vi "BucketNearMatchingPngFiles.vi"(10 "All PNG Files":path[](array[path])) -> (3 "All PNG Files (Bucketed by Near-Matches)":cluster{"Similar PNG Files":path[]}[](array[cluster]))   [LabVIEW 2020]
panel:
  out "Image buckets":i32[](array[numeric])
  out "Report":string
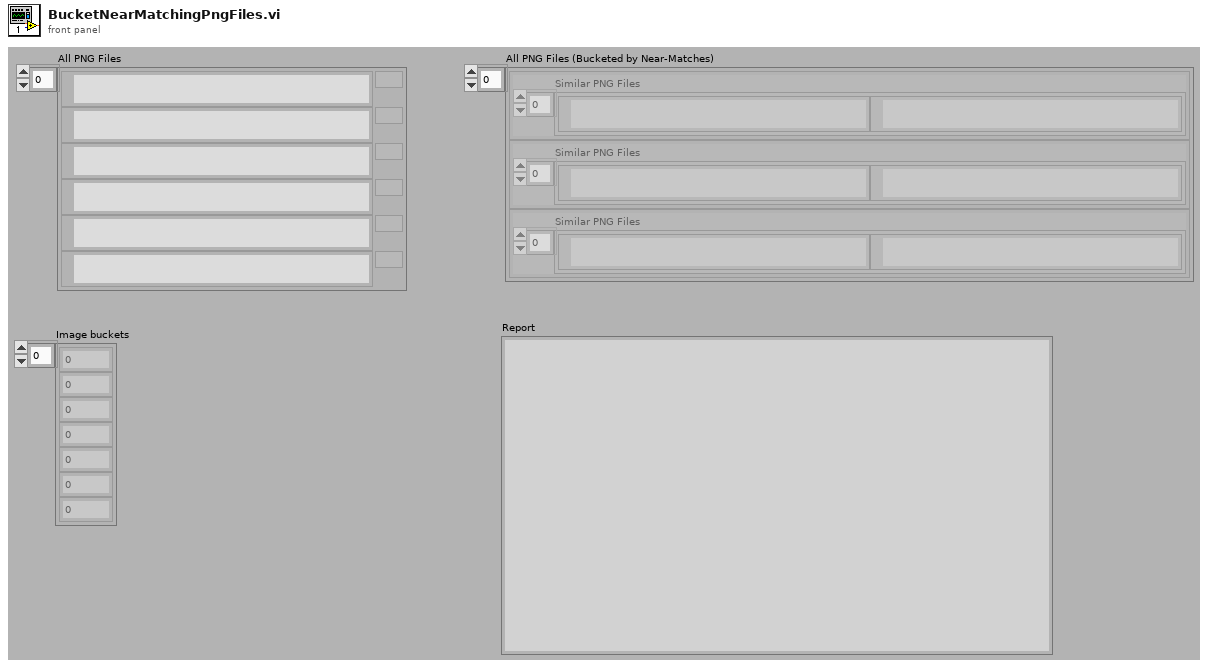
[diagram p1: front panel]
types:
  T1 = typedef "imagedata.ctl" = cluster{"image type":i32, "image depth":i32, "image":u8[], "mask":u8[], "colors":u32[], "Rectangle":cluster{"left":i16, "top":i16, "right":i16, "bottom":i16}}
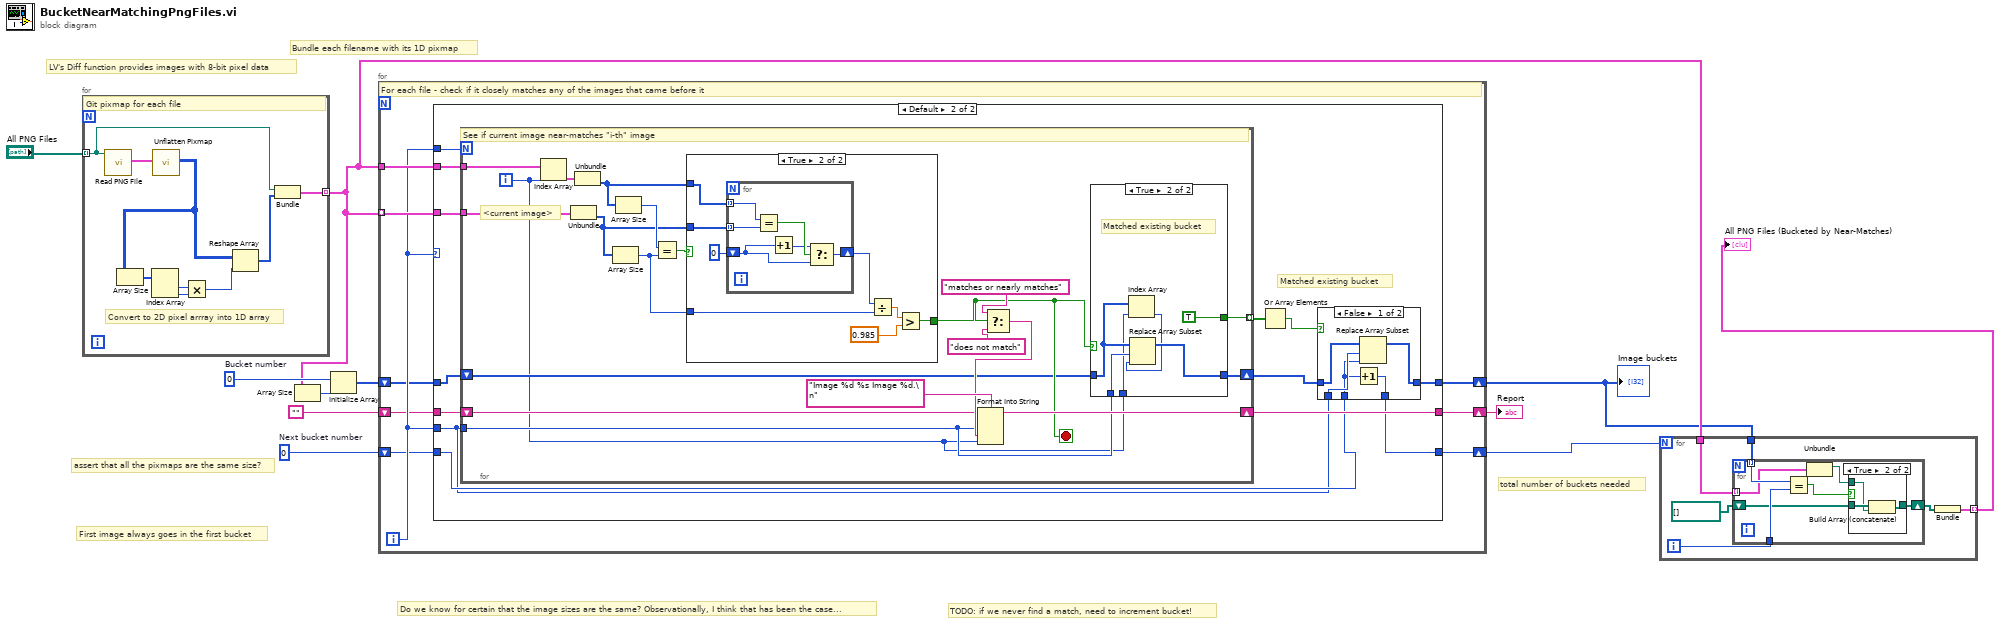
[diagram p0: block diagram]
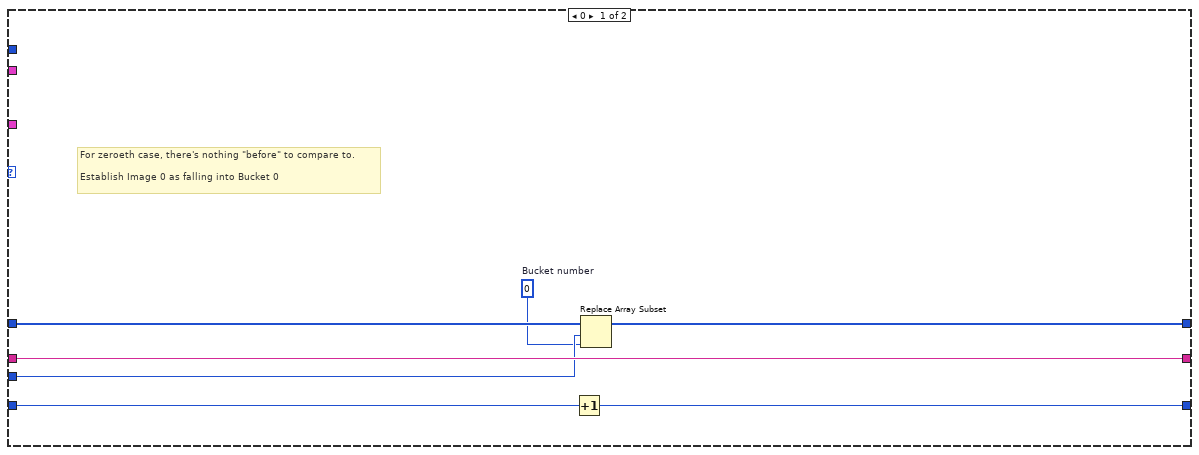
[diagram p3: hidden frame]
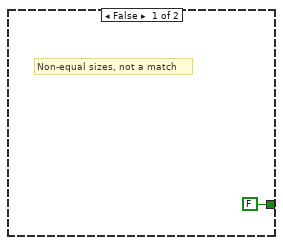
[diagram p6: hidden frame]
diagram:
  w5 = 0  # Next bucket number
  w8 = 0  # Bucket number
  # "total number of buckets needed"
  # "TODO: if we never find a match, need to increment bucket!"
  # "Do we know for certain that the image sizes are the same? Observationally, I think that has been the case..."
  # "Bundle each filename with its 1D pixmap"
  # "First image always goes in the first bucket"
  # "LV's Diff function provides images with 8-bit pixel data"
  # "assert that all the pixmaps are the same size?"
  n1 = for {
    tunnel: "All PNG Files" -> [w14] mode=indexing
    tunnel: [w12] -> w3 mode=indexing
    # "Convert to 2D pixel arrray into 1D array"
    # "Git pixmap for each file"
    n2 = call <vilib>:"Read PNG File.vi"("path to PNG file"=w14) -> ("image data"=w20:T1)  [unwired: 8 in, 2 out]
    n3 = call <vilib>:"Unflatten Pixmap.vi"("image data"=w20) -> ("8-bit pixmap"=w15:u8[][])  [unwired: 4 in, 6 out]
    n4 = Array Size(array=w15) -> (size(s)=w19:i32[])
    n5 = Index Array(array=w19) -> (element #1=w17:i32, element #2=w18:i32)  [unwired: 2 in]
    n6 = Multiply(x=w17, y=w18) -> (x*y=w16:i32)
    n7 = Reshape Array(w15, w16) -> (w13:u8[])
    n8 = Bundle("Path"=w14, "8-bit pixmap"=w13) -> (w12:cluster{"Path":path, "8-bit pixmap":u8[]})  [unwired: 1 in]
  }
  n9 = Array Size(array=w3) -> (size(s)=w7:i32)
  n10 = Initialize Array(w8, w7) -> (w6:i32[])
  n11 = for {
    tunnel: w3 -> [w29] mode=indexing
    tunnel: w3 -> [w28]
    shift-right: [w25] -> w9
    shift-left: "" -> [w26]
    shift-right: [w23] -> w2
    shift-left: w6 -> [w24]
    shift-right: [w21] -> w4
    shift-left: w5 -> [w22]
    i -> [w27]
    # "For each file - check if it closely matches any of the images that came before it"
    n12 = case shown="Default" w27 {
      tunnel: w27 -> [_ w49]
      tunnel: w29 -> [_ w48]
      tunnel: w28 -> [_ w47]
      tunnel: w27 -> [w33 w37]
      tunnel: w26 -> [w36 w46]
      tunnel: [w36 w45] -> w25
      tunnel: w24 -> [w35 w44]
      tunnel: [w34 w41] -> w23
      tunnel: w22 -> [w31 w39]
      tunnel: [w30 w38] -> w21
      frame 0 {
        w32 = 0  # Bucket number
        # "For zeroeth case, there's nothing \"before\" to compare to.\n\nEstablish Image 0 as falling into Bucket 0"
        n13 = Increment(x=w31) -> (x+1=w30:i32)
        n14 = Replace Array Subset(array=w35, new element=w32, index=w33) -> (w34:i32[])
      }
      frame Default {
        # "Matched existing bucket"
        n15 = for {
          N: w49 -> [_]
          tunnel: w48 -> [w74]
          tunnel: w47 -> [w76]
          tunnel: w37 -> [w59]
          shift-right: [w63] -> w45
          shift-left: w46 -> [w64]
          shift-right: [w60] -> w40
          shift-left: w44 -> [w61]
          tunnel: [w57] -> w43 mode=indexing
          i -> [w58]
          stop <- w62 stop-if-true
          # "<current image>"
          # "See if current image near-matches \"i-th\" image"
          n16 = Index Array(array=w76, index=w58) -> (element=w75:cluster{"Path":path, "8-bit pixmap":u8[]})
          n17 = Unbundle(w74) -> ("8-bit pixmap"=w70:u8[])  [unwired: 1 out]
          n18 = Unbundle(w75) -> ("8-bit pixmap"=w71:u8[])  [unwired: 1 out]
          n19 = Array Size(array=w70) -> (size(s)=w69:i32)
          n20 = Array Size(array=w71) -> (size(s)=w73:i32)
          n21 = Equal?(x=w73, y=w69) -> (x = y?=w72:bool)
          n22 = case shown="True" w72 {
            tunnel: w71 -> [_ w92]
            tunnel: w70 -> [_ w91]
            tunnel: w69 -> [_ w89]
            tunnel: [FALSE w85] -> w62
            frame False {
              # "Non-equal sizes, not a match"
            }
            frame True {
              n23 = for {
                tunnel: w92 -> [w97] mode=indexing
                tunnel: w91 -> [w98] mode=indexing
                shift-right: [w96] -> w88
                shift-left: 0 -> [w93]
                n24 = Equal?(x=w97, y=w98) -> (x = y?=w95:bool)
                n25 = Increment(x=w93) -> (x+1=w94:i32)
                n26 = Select(t=w94, s=w95, f=w93) -> (s? t:f=w96:i32)
              }
              n27 = Divide(x=w88, y=w89) -> (x/y=w87:dbl)
              n28 = Greater?(x=w87, y=0.985) -> (0:w85:bool)
            }
          }
          n29 = Select(t="matches or nearly matches", s=w62, f="does not match") -> (s? t:f=w65:string)
          n30 = Format Into String(format string="Image %d %s Image %d.\n", initial string=w64, w59, w65, w58) -> (resulting string=w63:string)  [unwired: 1 in, 1 out]
          n31 = case shown="True" w62 {
            tunnel: w61 -> [w77 w81]
            tunnel: [w77 w83] -> w60
            tunnel: w59 -> [_ w82]
            tunnel: w58 -> [_ w80]
            tunnel: [_ TRUE] -> w57
            frame False {
            }
            frame True {
              # "Matched existing bucket"
              n32 = Index Array(array=w81, index=w80) -> (element=w79:i32)
              n33 = Replace Array Subset(array=w81, new element=w79, index=w82) -> (w83:i32[])
            }
          }
        }
        n34 = Or Array Elements(Boolean array=w43) -> (logical OR=w42:bool)
        n35 = case shown="False" w42 {
          tunnel: [w53 w56] -> w41
          tunnel: w40 -> [w54 w56]
          tunnel: w39 -> [w51 w55]
          tunnel: [w50 w55] -> w38
          tunnel: w37 -> [w52 _]
          frame False {
            n36 = Increment(x=w51) -> (x+1=w50:i32)
            n37 = Replace Array Subset(array=w54, new element=w51, index=w52) -> (w53:i32[])
          }
          frame True {
          }
        }
      }
    }
  }
  "Report" <- w9
  "Image buckets" <- w2
  n38 = for {
    N: w4 -> [_]
    tunnel: w3 -> [w104]
    tunnel: w2 -> [w103]
    tunnel: [w99] -> w1 mode=indexing
    i -> [w102]
    n39 = for {
      tunnel: w104 -> [w109] mode=indexing
      tunnel: w103 -> [w110] mode=indexing
      tunnel: w102 -> [w111]
      shift-right: [w106] -> w100
      shift-left: path[] [] ("Similar PNG Files") -> [w105]
      n40 = Equal?(x=w110, y=w111) -> (x = y?=w108:bool)
      n41 = Unbundle(w109) -> ("Path"=w107:path)  [unwired: 1 out]
      n42 = case shown="True" w108 {
        tunnel: w107 -> [_ w114]
        tunnel: [w112 w113] -> w106
        tunnel: w105 -> [w112 w115]
        frame False {
        }
        frame True {
          n43 = Build Array (concatenate)(w115, w114) -> (w113:path[])
        }
      }
    }
    n44 = Bundle("Similar PNG Files"=w100) -> (w99:cluster{"Similar PNG Files":path[]})  [unwired: 1 in]
  }
  "All PNG Files (Bucketed by Near-Matches)" <- w1
